vi "Vtest.vi"() -> ()   [LabVIEW 2024]
uses:
  <vilib>/Analysis/baseanly.llb/Mean (DBL).vi
  <instrlib>/EFmeter/EFmeter.lvlib
  <vilib>/Analysis/NI_AALBase.lvlib
  BK Precision 8500B Series/BK Precision 8500B Series.lvlib
  Keithley 2200 Series/Keithley 2200 Series.lvlib
  Keithley DMM6500 DAQ6500 Series.lvlib
panel:
  in  "VISA DMM":refnum<visa-resource-name>
  in  "Zdroj":u16(ring) items=["Manualni", "K 2200"]
  out "error out 2":errorcluster
  in  "VISA EFmeter":refnum<visa-resource-name>
  out "R_out":dbl
  in  "file path (use dialog)":path
  in  "Prodleva mezi vzorky":u32
  out "napeti":dbl=2.5
  in  "velikost kroku":dbl
  in  "start":dbl
  in  "Prumerovani":bool
  in  "Vzorku na krokù":u16 max=100 step=1
  out "XY Graph 2":cluster{"X":dbl[], "Y":dbl[]}[](graph)
  in  "Pocet kroku":i32
  in  "Clear":bool
  in  "Uložit data":bool
  in  "Start":bool
  in  "VISA zdroj":refnum<visa-resource-name>
  in  "stop":bool
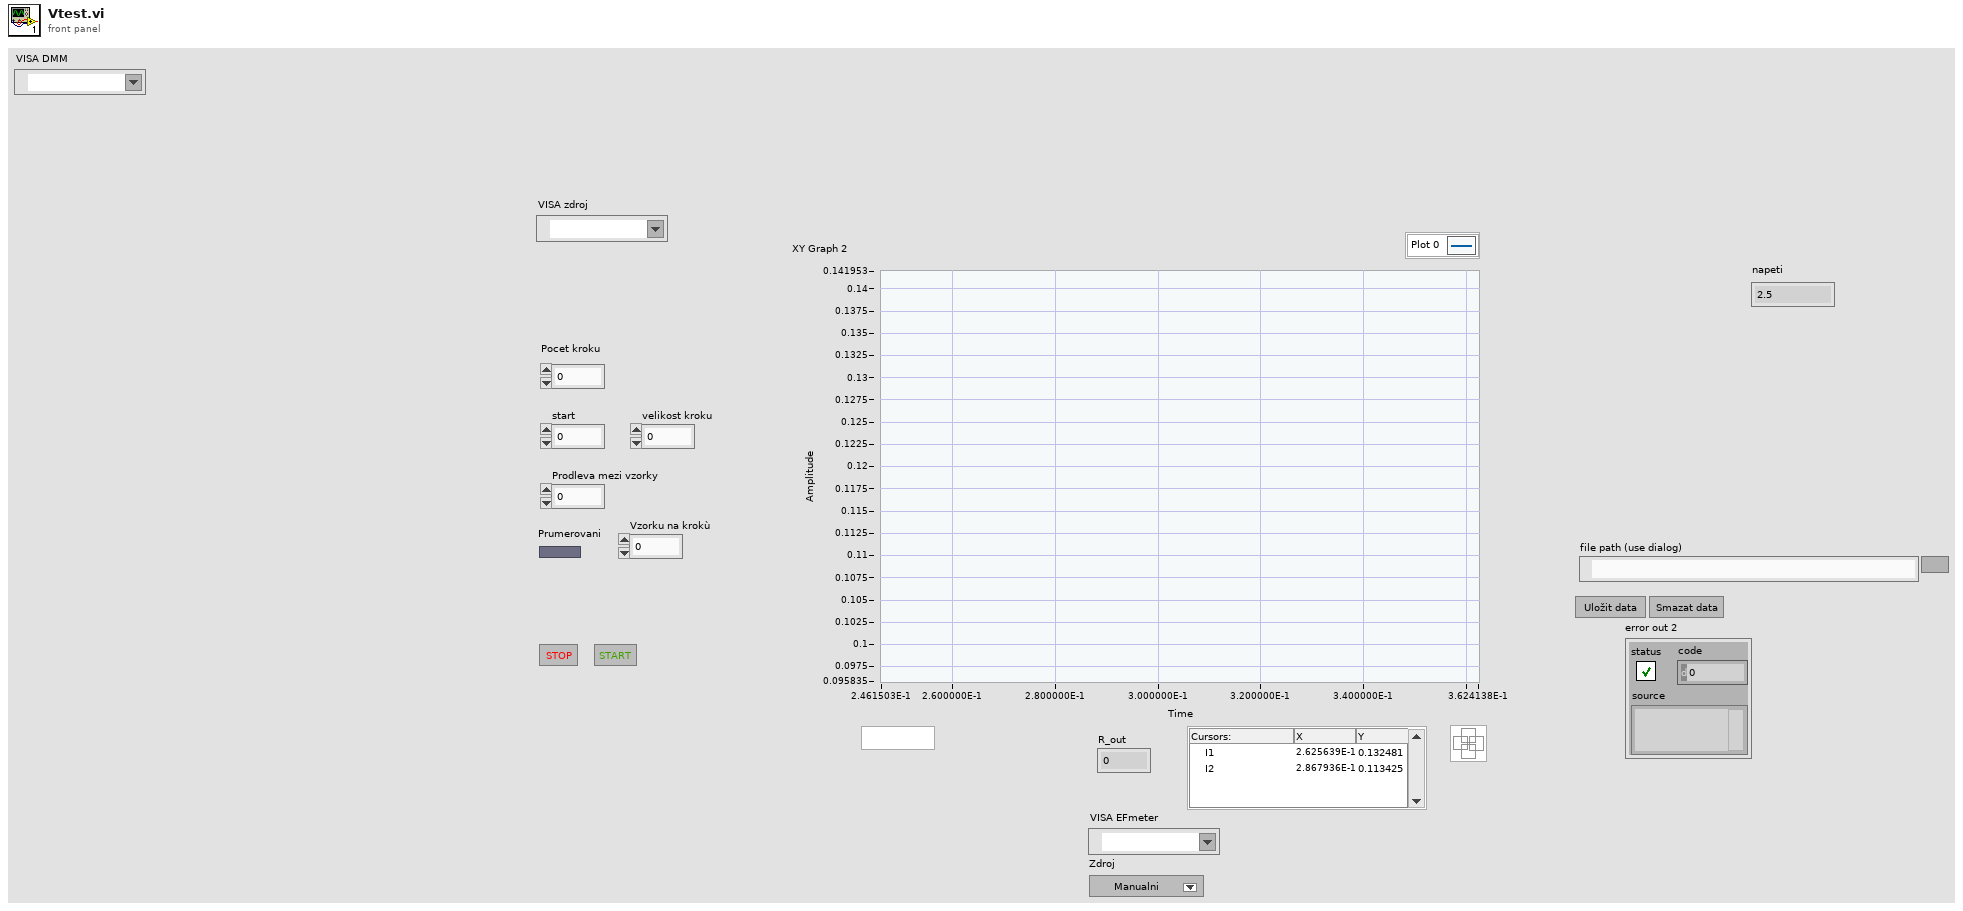
[diagram p1: front panel]
types:
  T1 = enum16{"init", "wait", "graph", "meas", "change_load", "init_measurment", "save", "clear"}
  T2 = typedef "LVCursorListTypeDef.ctl" = cluster{"Name":string, "Color":u32, "Style":u8, "Point Style":u8, "Name Visible":bool, "Allow Drag":bool, "Cursor Mode":u32, "Plot":i32, "Index":i32, "Position":cluster{"X":dbl, "Y":dbl}, "X Scale":u32, "Y Scale":u32, "Watch Plots":i32[], "Watch All Plots":bool, "Plot Area":i32, "Label Offset":cluster{"X":dbl, "Y":dbl}}[]
  T3 = cluster{"Name":string, "Color":u32, "Style":u8, "Point Style":u8, "Name Visible":bool, "Allow Drag":bool, "Cursor Mode":u32, "Plot":i32, "Index":i32, "Position":cluster{"X":dbl, "Y":dbl}, "X Scale":u32, "Y Scale":u32, "Watch Plots":i32[], "Watch All Plots":bool, "Plot Area":i32, "Label Offset":cluster{"X":dbl, "Y":dbl}}
  T4 = enum16{"open", "replace", "create", "open or create", "replace or create", "replace or create with confirmation"}
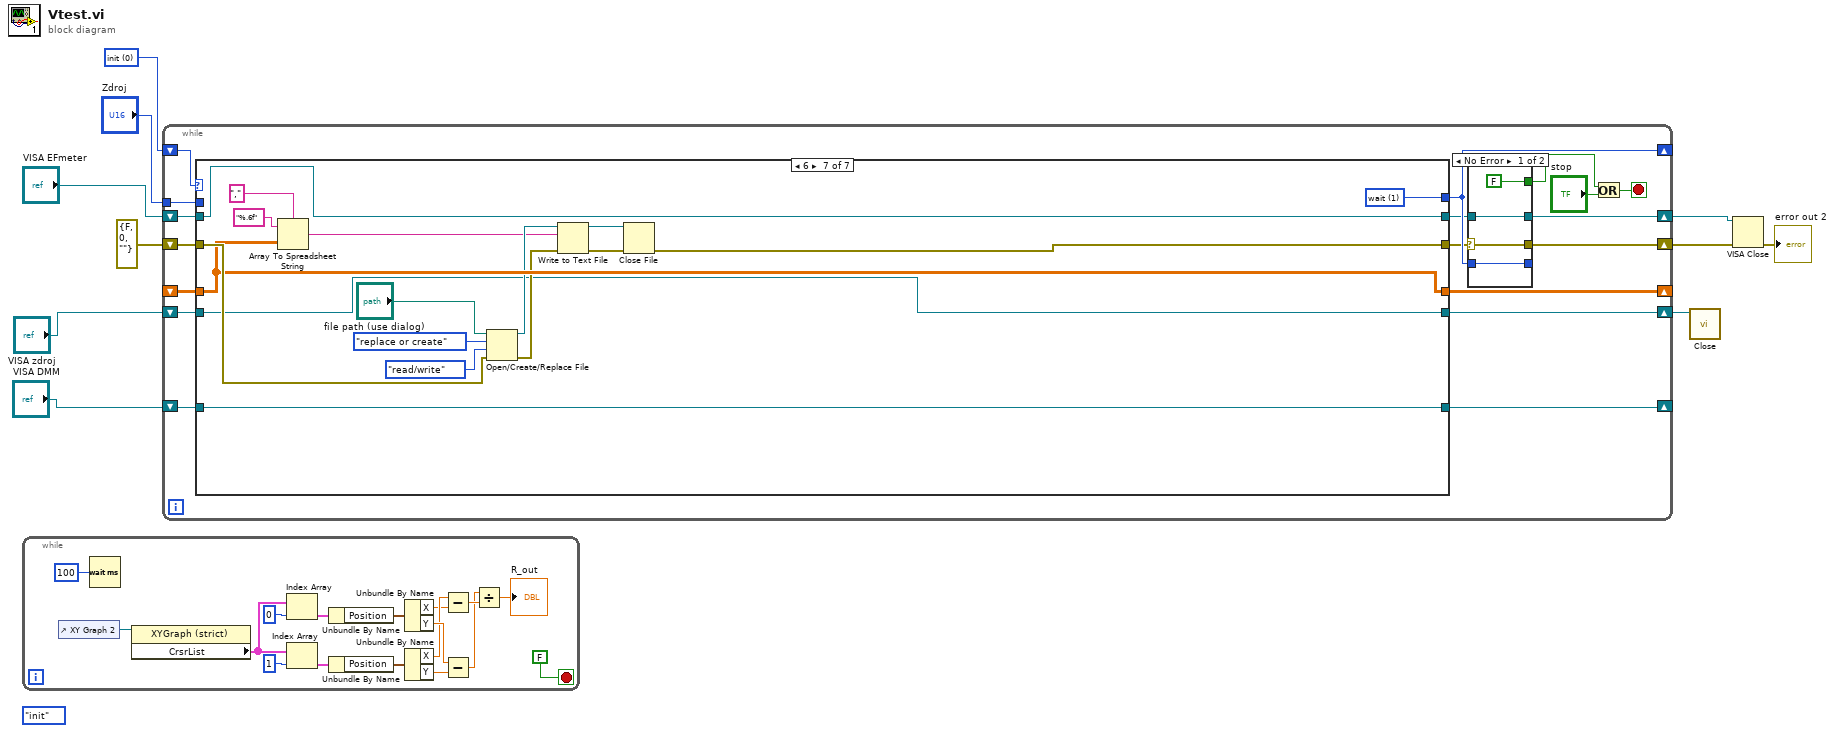
[diagram p0: block diagram]
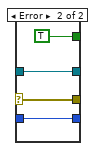
[diagram p2: hidden frame]
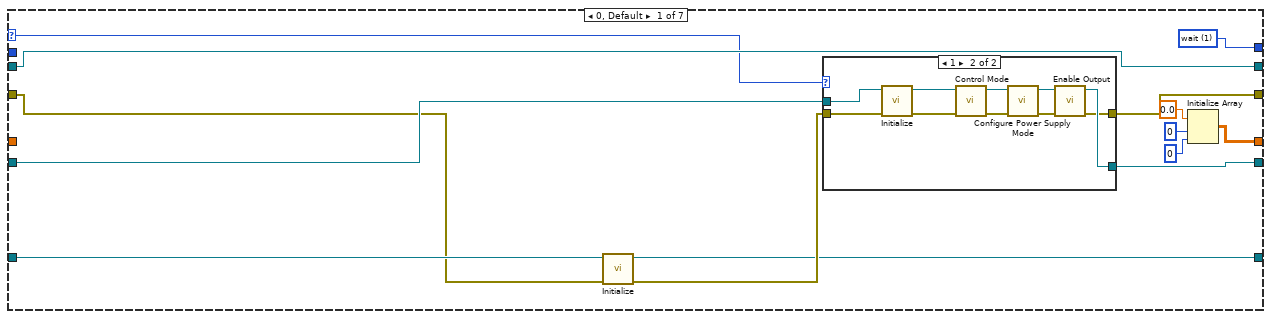
[diagram p3: hidden frame]
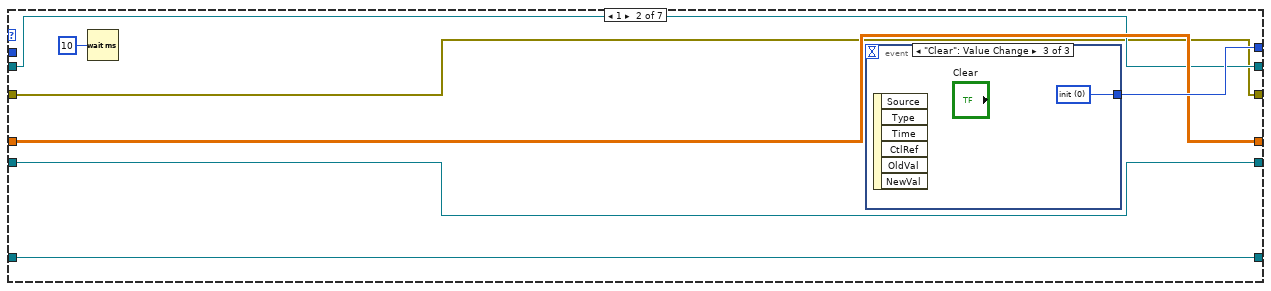
[diagram p5: hidden frame]
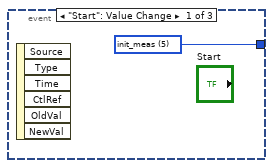
[diagram p6: hidden frame]
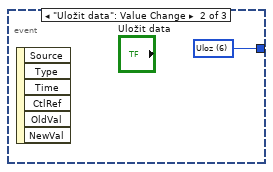
[diagram p7: hidden frame]
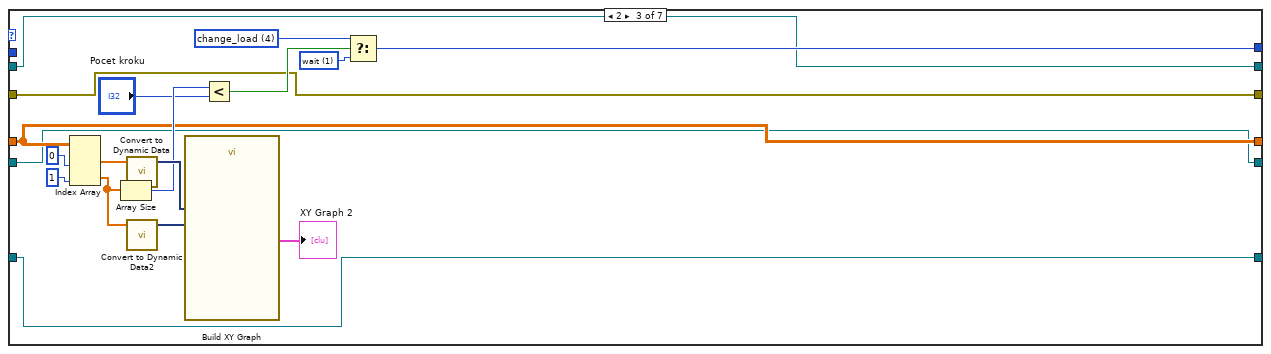
[diagram p8: hidden frame]
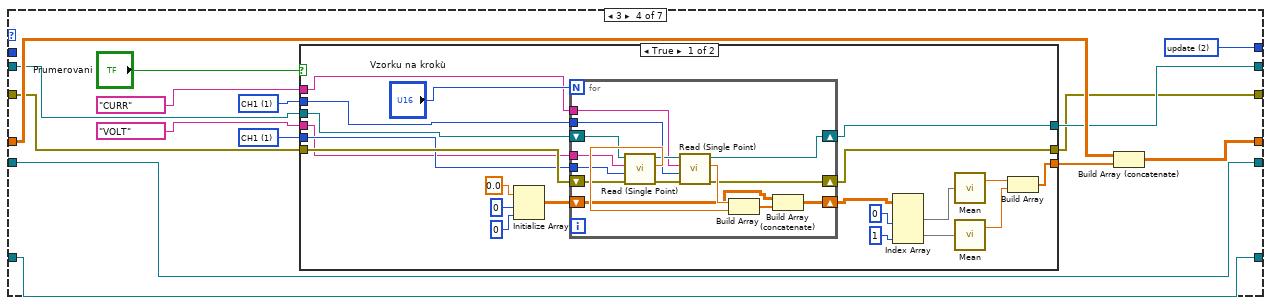
[diagram p9: hidden frame]
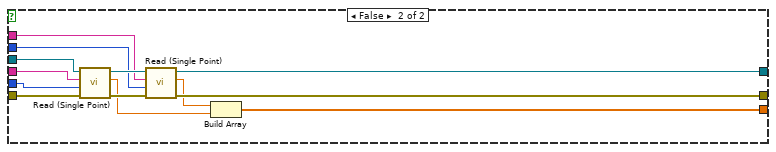
[diagram p10: hidden frame]
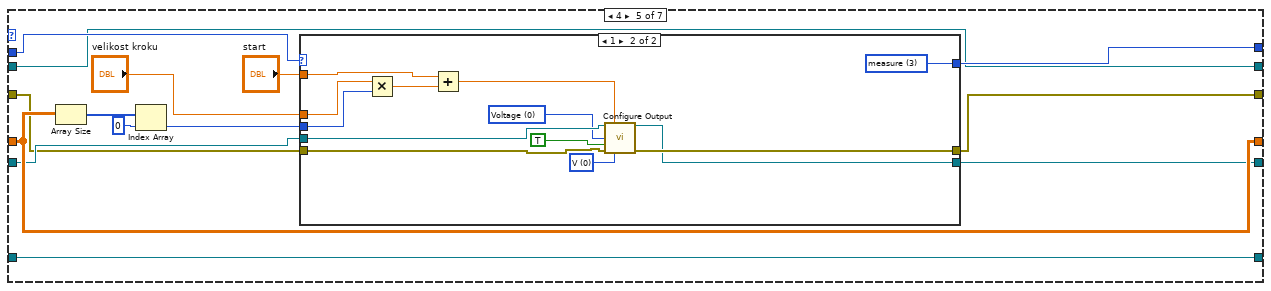
[diagram p11: hidden frame]
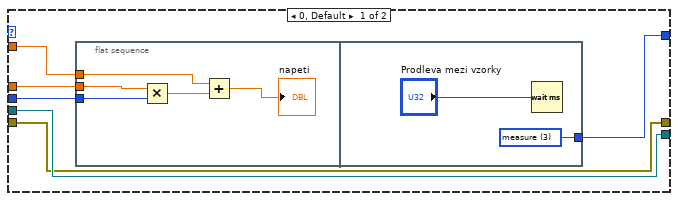
[diagram p12: hidden frame]
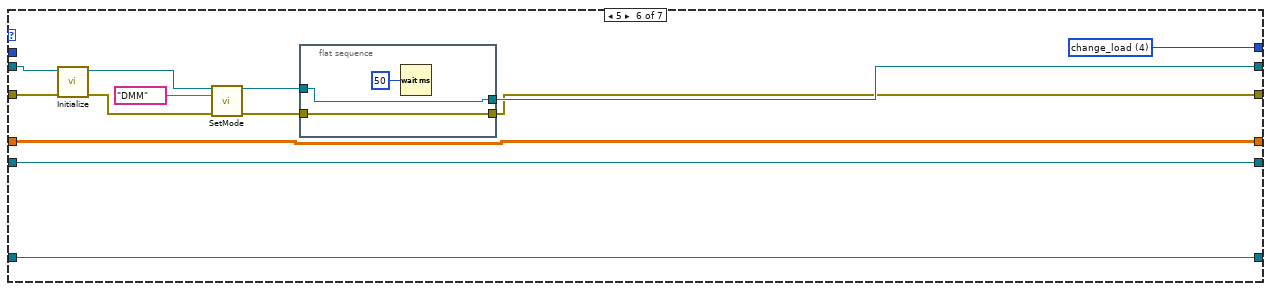
[diagram p13: hidden frame]
diagram:
  (unwired) T1."init"
  w10 = u16 0 items=["init", "wait", "update", "measure", "change_load", "init_meas", "Uloz", "clear"]
  n1 = while {
    stop <- FALSE stop-if-true
    n2 = control-ref of="XY Graph 2"() -> (w25:refnum<vi>)
    n3 = Wait (ms)(milliseconds to wait=u32 100) -> ()  [unwired: 1 out]
    n4 = property class="XYGraph (strict)"(reference=w25) -> ("CrsrList"=w20:T2)  [unwired: 1 in, 2 out]
    n5 = Index Array(array=w20, index=0) -> (element=w26:T3)
    n6 = Index Array(array=w20, index=1) -> (element=w22:T3)
    n7 = Unbundle By Name(w26) -> ("Position"=w27:cluster{"X":dbl, "Y":dbl})
    n8 = Unbundle By Name(w22) -> ("Position"=w23:cluster{"X":dbl, "Y":dbl})
    n9 = Unbundle By Name(w27) -> ("X"=w11:dbl, "Y"=w18:dbl)
    n10 = Unbundle By Name(w23) -> ("X"=w12:dbl, "Y"=w19:dbl)
    n11 = Subtract(x=w12, y=w11) -> (x-y=w14:dbl)
    n12 = Subtract(x=w18, y=w19) -> (x-y=w13:dbl)
    n13 = Divide(x=w13, y=w14) -> (x/y=→"R_out":dbl)
  }
  n14 = while {
    shift-right: [w45] -> _
    shift-left: _ -> [w44]
    shift-right: [w40] -> _
    shift-left: w10 -> [w43]
    shift-right: [w37] -> w6
    shift-left: "VISA EFmeter" -> [w42]
    shift-right: [w36] -> w5
    shift-left: errorcluster {"status"=FALSE, "code"=0, "source"=""} ("error in (no error)") -> [w41]
    tunnel: "Zdroj" -> [w32]
    shift-right: [w31] -> w3
    shift-left: "VISA zdroj" -> [w30]
    shift-right: [w28] -> _
    shift-left: "VISA DMM" -> [w29]
    stop <- w34 stop-if-true
    n15 = case shown="6" w43 {
      selector: w43 -> [w61 _ _ _ _ _ _]
      tunnel: [w65 w85 w99 w121 w185 w224 w239] -> w45
      tunnel: w44 -> [_ w85 w99 w122 w185 w224 w239]
      tunnel: [w64 w86 w98 w119 w183 w218 w237] -> w40
      tunnel: [w60 w83 w92 w111 w173 w215 w233] -> w39
      tunnel: [w62 w84 w93 w112 w182 w217 w244] -> w38
      tunnel: w42 -> [w62 w84 w93 w118 w182 w220 w244]
      tunnel: w41 -> [w56 w83 w92 w117 w174 w219 w240]
      tunnel: w32 -> [_ _ _ _ w184 _ _]
      tunnel: [w59 w81 w91 w109 w180 w213 w229] -> w31
      tunnel: w30 -> [w58 w81 w91 w109 w181 w213 w229]
      tunnel: w29 -> [w57 w80 w90 w108 w172 w212 w228]
      tunnel: [w54 w80 w90 w108 w172 w212 w228] -> w28
      frame 0, Default {
        w64 = u16 1 items=["init", "wait", "update", "measure"]
        n16 = call "Initialize.vi"("error in (no error)"=w56, "VISA resource name"=w57) -> ("error out"=w55:errorcluster, "VISA resource name out"=w54:refnum<visa-resource-name>)  [unwired: 8 in]
        n17 = case shown="1" w61 {
          tunnel: w55 -> [w69 w79]
          tunnel: [w69 w70] -> w60
          tunnel: [w68 w71] -> w59
          tunnel: w58 -> [w68 w78]
          frame 0, Default {
          }
          frame 1 {
            n18 = call "Initialize.vi"("error in (no error)"=w79, "VISA resource name"=w78) -> ("error out"=w77:errorcluster, "VISA resource name out"=w76:refnum<visa-resource-name>)  [unwired: 8 in]
            n19 = call "Control Mode.vi"("error in (no error)"=w77, "VISA resource name"=w76) -> ("error out"=w72:errorcluster, "VISA resource name out"=w73:refnum<visa-resource-name>)  [unwired: 8 in]
            n20 = call "Configure Power Supply Mode.vi"("error in (no error)"=w72, "VISA resource name"=w73) -> ("error out"=w75:errorcluster, "VISA resource name out"=w74:refnum<visa-resource-name>)  [unwired: 8 in]
            n21 = call "Enable Output.vi"("error in (no error)"=w75, "VISA resource name"=w74) -> ("error out"=w70:errorcluster, "VISA resource name out"=w71:refnum<visa-resource-name>)  [unwired: 8 in]
          }
        }
        n22 = Initialize Array(0.0 ("element"), 0 ("dimension size"), 0 ("dimension size")) -> (w65:dbl[][])
      }
      frame 1 {
        n23 = Wait (ms)(milliseconds to wait=u32 10) -> ()  [unwired: 1 out]
        n24 = event shown="[2] \"Clear\": Value Change" {
          selector: _ -> [_ _ _]
          dyn-events: _ -> [_ _ _]
          timeout: _ -> [_ _ _]
          tunnel: [w87 w88 w89] -> w86
          event "Start": Value Change {
            w87 = u16 5 items=["init", "wait", "update", "measure", "change_load", "init_meas"]
            n25 = event-data() -> ()  [unwired: 1 in, 6 out]
          }
          event "Uložit data": Value Change {
            w88 = u16 6 items=["init", "wait", "update", "measure", "change_load", "init_meas", "Uloz"]
            n26 = event-data() -> ()  [unwired: 1 in, 6 out]
          }
          event "Clear": Value Change {
            w89 = u16 0 items=["init", "wait", "update", "measure", "change_load", "init_meas", "Uloz", "clear"]
            n27 = event-data() -> ()  [unwired: 1 in, 6 out]
          }
        }
      }
      frame 2 {
        w94 = u16 4 items=["init", "wait", "update", "measure", "change_load", "init_meas"]
        w100 = u16 1 items=["init", "wait", "update", "measure"]
        n28 = Index Array(array=w99, index (col) #1=0 ("index (row)"), index (col) #2=1 ("index (row)")) -> (element #1=w107:dbl[], element #2=w102:dbl[])  [unwired: 2 in]
        n29 = Array Size(array=w102) -> (size(s)=w104:i32)
        n30 = call "Convert to Dynamic Data"("Array"=w107) -> ("Dynamic Data Type"=w106:dynamicdata)  [unwired: 3 in]
        n31 = call "Convert to Dynamic Data2"("Array"=w102) -> ("Dynamic Data Type"=w105:dynamicdata)  [unwired: 3 in]
        n32 = call "Build XY Graph"("Y Input"=w105, "X Input"=w106) -> ("XY Graph"=→"XY Graph 2":cluster{"X":dbl[], "Y":dbl[]}[])  [unwired: 8 in, 1 out]
        n33 = Less?(x=w104, y="Pocet kroku") -> (x < y?=w103:bool)
        n34 = Select(t=w94, s=w103, f=w100) -> (s? t:f=w98:u16)
      }
      frame 3 {
        w113 = u16 1 items=["CH2"=2, "CH1"=1] ("Ring")
        w116 = u16 1 items=["CH2"=2, "CH1"=1] ("Ring")
        w119 = u16 2 items=["init", "wait", "update", "measure"]
        n35 = case shown="True" "Prumerovani" {
          tunnel: [w125 w171] -> w120
          tunnel: w118 -> [w138 w170]
          tunnel: w117 -> [w137 w169]
          tunnel: w116 -> [w136 w168]
          tunnel: "VOLT" ("Combo Box") -> [w135 w167]
          tunnel: "CURR" ("Combo Box") -> [w134 w164]
          tunnel: w113 -> [w133 w163]
          tunnel: [w124 w162] -> w112
          tunnel: [w123 w161] -> w111
          frame True {
            n36 = Initialize Array(0.0 ("element"), 0 ("dimension size"), 0 ("dimension size")) -> (w139:dbl[][])
            n37 = for {
              N: "Vzorku na krokù" -> [_]
              shift-right: [w151] -> w124
              shift-left: w138 -> [w152]
              shift-right: [w149] -> w123
              shift-left: w137 -> [w150]
              tunnel: w136 -> [w148]
              tunnel: w135 -> [w147]
              tunnel: w134 -> [w146]
              tunnel: w133 -> [w145]
              shift-right: [w144] -> w132
              shift-left: w139 -> [w153]
              n38 = call "Read (Single Point).vi"("error in (no error)"=w150, "Ring"=w148, "Combo Box"=w147, "VISA resource name"=w152) -> ("error out"=w156:errorcluster, "Measurement"=w158:dbl, "VISA resource name out"=w157:refnum<visa-resource-name>)  [unwired: 5 in]
              n39 = call "Read (Single Point).vi"("error in (no error)"=w156, "Ring"=w145, "Combo Box"=w146, "VISA resource name"=w157) -> ("error out"=w149:errorcluster, "Measurement"=w155:dbl, "VISA resource name out"=w151:refnum<visa-resource-name>)  [unwired: 5 in]
              n40 = Build Array(w155, w158) -> (w154:dbl[])
              n41 = Build Array (concatenate)(w153, w154) -> (w144:dbl[][])
            }
            n42 = Index Array(array=w132, index (col) #1=0 ("disabled index (col)"), index (col) #2=1 ("index (col)")) -> (element #1=w131:dbl[], element #2=w130:dbl[])  [unwired: 2 in]
            n43 = call-poly <vilib>:"Mean.vi"("X"=w131) -> ("mean"=w127:dbl)  [unwired: 1 out]
            n44 = call-poly <vilib>:"Mean.vi"("X"=w130) -> ("mean"=w126:dbl)  [unwired: 1 out]
            n45 = Build Array(w127, w126) -> (w125:dbl[])
          }
          frame False {
            n46 = call "Read (Single Point).vi"("error in (no error)"=w169, "Ring"=w168, "Combo Box"=w167, "VISA resource name"=w170) -> ("error out"=w166:errorcluster, "Measurement"=w159:dbl, "VISA resource name out"=w165:refnum<visa-resource-name>)  [unwired: 5 in]
            n47 = call "Read (Single Point).vi"("error in (no error)"=w166, "Ring"=w163, "Combo Box"=w164, "VISA resource name"=w165) -> ("error out"=w161:errorcluster, "Measurement"=w160:dbl, "VISA resource name out"=w162:refnum<visa-resource-name>)  [unwired: 5 in]
            n48 = Build Array(w160, w159) -> (w171:dbl[])
          }
        }
        n49 = Build Array (concatenate)(w122, w120) -> (w121:dbl[][])
      }
      frame 4 {
        n50 = Array Size(array=w185) -> (size(s)=w175:i32[])
        n51 = Index Array(array=w175, index=0) -> (element=w177:i32)
        n52 = case shown="1" w184 {
          tunnel: [w191 w211] -> w183
          tunnel: w181 -> [w190 w202]
          tunnel: [w190 w201] -> w180
          tunnel: "velikost kroku" -> [w189 w209]
          tunnel: "start" -> [w188 w207]
          tunnel: w177 -> [w187 w210]
          tunnel: w174 -> [w186 w205]
          tunnel: [w186 w204] -> w173
          frame 0, Default {
            n53 = flat-sequence {
              tunnel: w189 -> [w194]
              tunnel: w188 -> [w193]
              tunnel: w187 -> [w192]
              tunnel: [w197] -> w191
              frame #0 {
                n54 = Multiply(x=w194, y=w192) -> (x*y=w196:dbl)
                n55 = Add(x=w193, y=w196) -> (x+y=→"napeti":dbl)
              }
              frame #1 {
                w197 = u16 3 items=["init", "wait", "update", "measure", "change_load", "init_meas"]
                n56 = Wait (ms)(milliseconds to wait="Prodleva mezi vzorky") -> ()  [unwired: 1 out]
              }
            }
          }
          frame 1 {
            w200 = u16 0 items=["Voltage", "Current"] ("Function(0:Voltage)")
            w203 = u16 0 items=["V", "mV", "kV", "A", "mA"] ("Unit(V)")
            w211 = u16 3 items=["init", "wait", "update", "measure", "change_load", "init_meas"]
            n57 = Multiply(x=w209, y=w210) -> (x*y=w208:dbl)
            n58 = Add(x=w207, y=w208) -> (x+y=w206:dbl)
            n59 = call "Configure Output.vi"("VISA resource name"=w202, "Manual Range(0.00)"=w206, "Function(0:Voltage)"=w200, "Enable Output (T: Enable)"=TRUE, "error in (no error)"=w205, "Unit(V)"=w203) -> ("VISA resource name out"=w201:refnum<visa-resource-name>, "error out"=w204:errorcluster)  [unwired: 8 in]
          }
        }
      }
      frame 5 {
        w218 = u16 4 items=["init", "wait", "update", "measure", "change_load", "init_meas"]
        n60 = call "Initialize.vi"("error in (no error)"=w219, "VISA resource name"=w220) -> ("error out"=w223:errorcluster, "VISA resource name out"=w222:refnum<visa-resource-name>)  [unwired: 8 in]
        n61 = call "SetMode.vi"("VISA resource name"=w222, "Combo Box"="DMM", "error in (no error)"=w223) -> ("VISA resource name out"=w216:refnum<visa-resource-name>, "error out"=w214:errorcluster)  [unwired: 11 in]
        n62 = flat-sequence {
          tunnel: [w226] -> w217
          tunnel: w216 -> [w226]
          tunnel: w214 -> [w225]
          tunnel: [w225] -> w215
          frame #0 {
            n63 = Wait (ms)(milliseconds to wait=u32 50) -> ()  [unwired: 1 out]
          }
        }
      }
      frame 6 {
        w237 = u16 1 items=["init", "wait", "update", "measure", "change_load", "init_meas"]
        n64 = Array To Spreadsheet String(delimiter (Tab)=",", array=w239, 3:"%.6f" ("format string")) -> (spreadsheet string=w230:string)
        n65 = Open/Create/Replace File(file path (use dialog)="file path (use dialog)", error in=w240, operation (0:open)=T4."replace or create", access (0:read/write)=enum16{"read/write", "read-only", "write-only"}."read/write") -> (refnum out=w232:refnum<file>, error out=w235:errorcluster)  [unwired: 2 in, 1 out]
        n66 = Write to Text File(file (use dialog)=w232, text=w230, error in=w235) -> (refnum out=w231:refnum<file>, error out=w234:errorcluster)  [unwired: 1 in, 1 out]
        n67 = Close File(refnum=w231, error in=w234) -> (error out=w233:errorcluster)  [unwired: 1 out]
      }
    }
    n68 = case shown="No Error" w39 {
      selector: w39 -> [w47 w51]
      tunnel: w40 -> [w49 w52]
      tunnel: [w49 w52] -> _
      tunnel: w38 -> [w48 w53]
      tunnel: [w48 w53] -> w37
      tunnel: [w47 w51] -> w36
      tunnel: [FALSE TRUE] -> w33
      frame No Error {
      }
      frame Error {
      }
    }
    n69 = Or(x=w33, y="stop") -> (x .or. y?=w34:bool)
  }
  n70 = call "Close.vi"("VISA resource name"=w3) -> ()  [unwired: 10 in, 1 out]
  n71 = VISA Close(VISA resource name=w6, error in (no error)=w5) -> (error out=→"error out 2":errorcluster)
